vi "WSVCAP SHL Host TL RFFE Read - Single DUT.vi"(0 "Data Out":string, 11 "error in":errorcluster, 12 "Log (T)":bool=TRUE, 13 "DUT":T1) -> (4 "Data In":string, 15 "error out":errorcluster)   [LabVIEW 2012]
uses:
  Type Defs/WSVCAP SHL DUT Number Enum.ctl
panel:
  out "RFFE Data In":u8[][](array[numeric]) format="%02x"
  out "Socket Mask":u64=1 format="%02x"
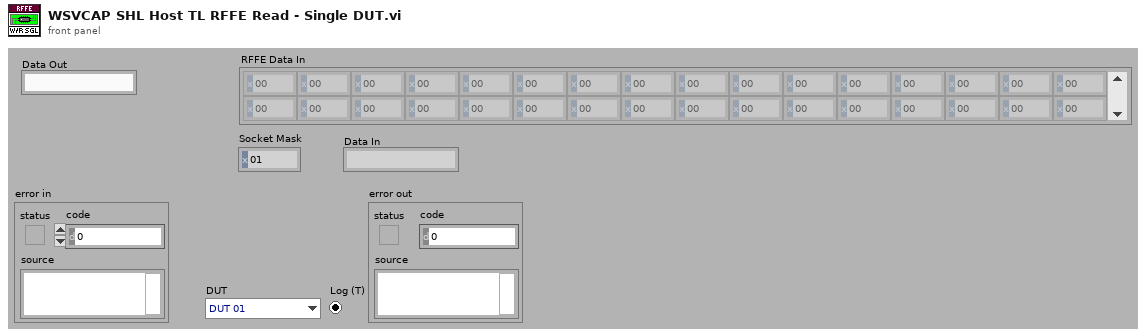
[diagram p1: front panel]
types:
  T1 = typedef "WSVCAP SHL DUT Number Enum.ctl" = enum16{"DUT 01", "DUT 02", "DUT 03", "DUT 04", "DUT 05", "DUT 06", "DUT 07", "DUT 08", "DUT 09", "DUT 10", "DUT 11", "DUT 12", "DUT 13", "DUT 14", "DUT 15", "DUT 16", "DUT 17", "DUT 18", "DUT 19", "DUT 20", "DUT 21", "DUT 22", "DUT 23", "DUT 24", "DUT 25", "DUT 26", "DUT 27", "DUT 28", "DUT 29", "DUT 30", "DUT 31", "DUT 32", "DUT 33", "DUT 34", "DUT 35", "DUT 36"}
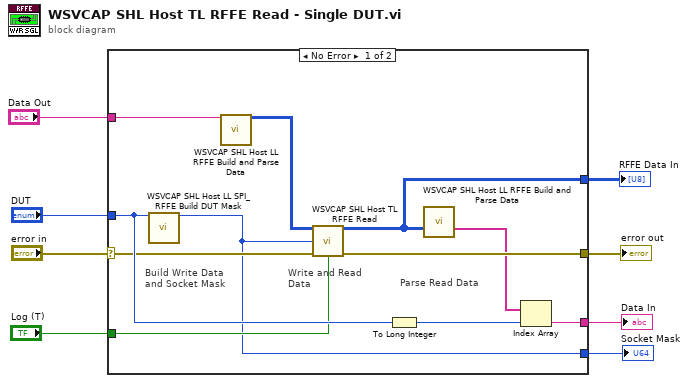
[diagram p0: block diagram]
diagram:
  n1 = case shown="No Error" "error in" {
    selector: "error in" -> [w18 _]
    tunnel: [w17 _] -> w8
    tunnel: "DUT" -> [w19 _]
    tunnel: [w15 _] -> w5
    tunnel: [w11 _] -> w4
    tunnel: [w12 _] -> w3
    tunnel: "Log (T)" -> [w14 _]
    tunnel: "Data Out" -> [w10 _]
    frame No Error {
      # "Parse Read Data"
      # "Write and Read\nData"
      # "Build Write Data and Socket Mask"
      n2 = call "WSVCAP SHL Host LL SPI_RFFE Build DUT Mask.vi"("DUT"=w19) -> ("Socket Mask [U64]"=w11:u64)  [unwired: 13 in, 1 out]
      n3 = call "WSVCAP SHL Host LL RFFE Build and Parse Data.vi"("Data Out"=w10) -> ("RFFE Data Out [U8]"=w9:u8[][])  [unwired: 11 in, 3 out]
      n4 = call "WSVCAP SHL Host TL RFFE Read.vi"("Write Data In [DUT Ordered]"=w9, "Socket Mask"=w11, "error in"=w18, "Log (T)"=w14) -> ("Read Data Out"=w12:u8[][], "error out"=w17:errorcluster)  [unwired: 10 in]
      n5 = To Long Integer(number=w19) -> (32bit integer=w16:i32)
      n6 = call "WSVCAP SHL Host LL RFFE Build and Parse Data.vi"("RFFE Data In [U8]"=w12) -> ("RFFE Data In"=w13:string[])  [unwired: 11 in, 3 out]
      n7 = Index Array(array=w13, index=w16) -> (element=w15:string)
    }
    frame Error {
    }
  }
  "error out" <- w8
  "Socket Mask" <- w4
  "Data In" <- w5
  "RFFE Data In" <- w3
